vi "H5Lcreate_external.vi"(4 "lcpl_id":T1, 6 "lapl_id":T1, 7 "Target Object Name":string, 8 "error in (no error)":errorcluster, 9 "Target File":path, 10 "Link Name":string, 11 "Link Location Ref":T1) -> (0 "error out":errorcluster, 3 "Link Location Ref out":T1)   [LabVIEW 2017]
doc: "Creates an external link, a soft link to an object in a different file."
uses:
  <vilib>/UPVI/lvhdf5/library.llb/HDF5 Ref.ctl
  <vilib>/UPVI/lvhdf5/hdf5.dll
panel:
  # "LVHDF5 Toolkit\nCopyright (c) 2005-2013 by Jason D. Sommerville\nCopyright (c) 2014-2015 by UPVI, LLC.\n\nThis use and distribution of this file is governed by the terms found in \nLICENSE.txt distributed with this toolkit and installed at\n <user.lib>\\_lvhdf5\\LICENSE.txt"
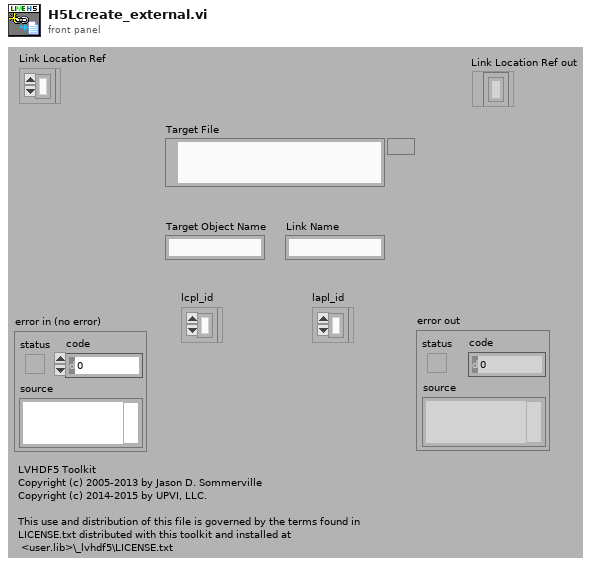
[diagram p1: front panel]
types:
  T1 = typedef "HDF5 Ref.ctl" = refnum<k1>
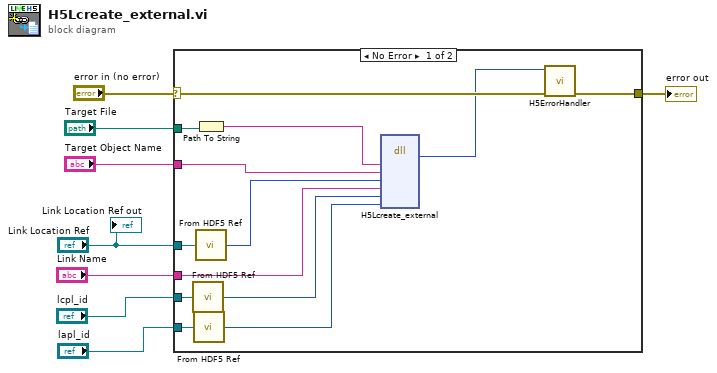
[diagram p0: block diagram]
diagram:
  n1 = case shown="No Error" "error in (no error)" {
    selector: "error in (no error)" -> [w21 w22]
    tunnel: [w20 w22] -> w7
    tunnel: "Link Location Ref" -> [w19 _]
    tunnel: "Target Object Name" -> [w9 _]
    tunnel: "Link Name" -> [w17 _]
    tunnel: "lcpl_id" -> [w16 _]
    tunnel: "lapl_id" -> [w15 _]
    tunnel: "Target File" -> [w11 _]
    frame No Error {
      n2 = call <vilib>:"From HDF5 Ref.vi"("HDF5 Ref"=w16) -> ("I32"=w14:i32)
      n3 = call <vilib>:"From HDF5 Ref.vi"("HDF5 Ref"=w15) -> ("I32"=w13:i32)
      n4 = Path To String(path=w11) -> (string=w10:string)
      n5 = call <vilib>:"From HDF5 Ref.vi"("HDF5 Ref"=w19) -> ("I32"=w12:i32)
      n6 = dll-call lib="C:/Program Files/National Instruments/LabVIEW 2017/vi.lib/UPVI/lvhdf5/hdf5.dll" fn="H5Lcreate_external" label="H5Lcreate_soft"("target_file_name"=w10, "target_obj_nam"=w9, "link_loc_id"=w12, "link_name"=w17, "lcpl_id"=w14, "lapl_id"=w13) -> ("return type"=w18:i32)  [unwired: 9 in, 2 out]
      n7 = call <vilib>:"H5ErrorHandler.vi"("error in (no error)"=w21, "herr_t"=w18) -> ("error out"=w20:errorcluster)  [unwired: 3 in, 4 out]
    }
    frame Error {
    }
  }
  "error out" <- w7
  "Link Location Ref out" <- "Link Location Ref"
